vi "LABVIWE_CALCULATOR_FORMULA_NODE.vi"() -> ()   [LabVIEW 2020]
panel:
  out "deivision":dbl
  out "Multiplication":dbl
  out "substraction":dbl
  out "addition":dbl
  in  "number  2":dbl
  in  "number1":dbl
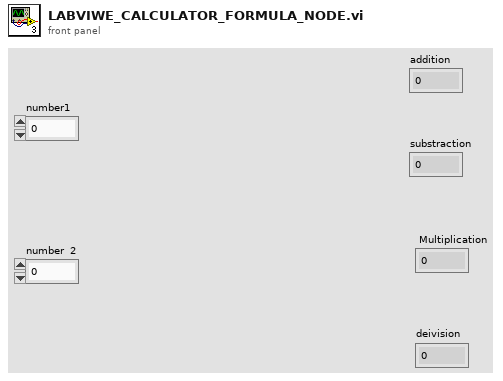
[diagram p1: front panel]
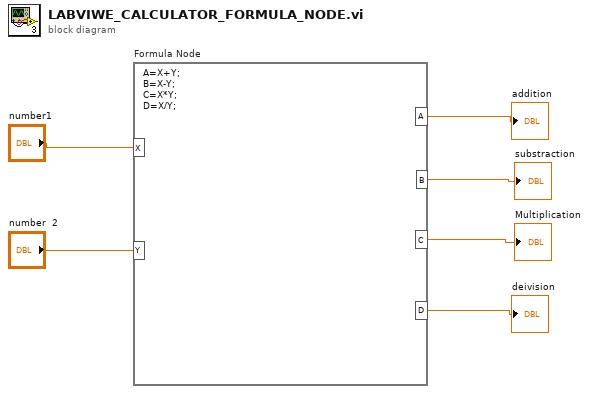
[diagram p0: block diagram]
diagram:
  n1 = formula code="A=X+Y;\nB=X-Y;\nC=X*Y;\nD=X/Y;"("X"="number1", "Y"="number  2") -> ("A"=→"addition":dbl, "B"=→"substraction":dbl, "C"=→"Multiplication":dbl, "D"=→"deivision":dbl)
